vi "stations PING.vi"(5 "error in (no error)":errorcluster, 7 "Ping Timeout (ms)":i32=5000, 8 "IP Address":string) -> (0 "error out":errorcluster, 1 "Valid Test Station?":bool, 3 "PING Response":string)   [LabVIEW 2011]
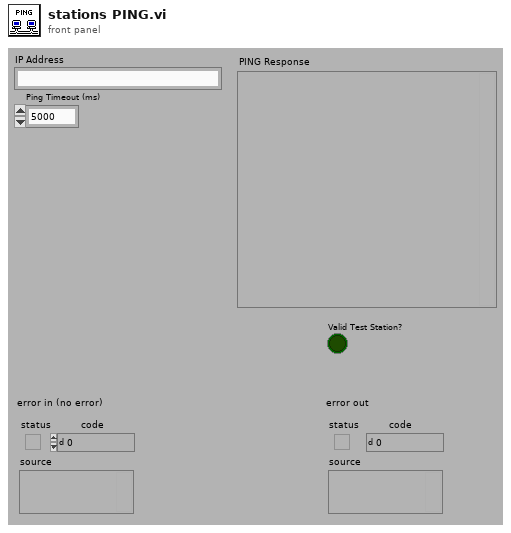
[diagram p1: front panel]
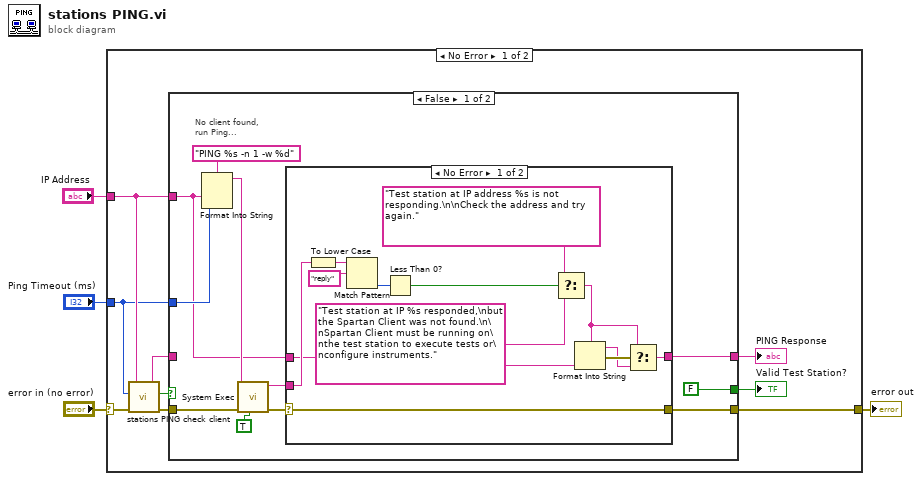
[diagram p0: block diagram]
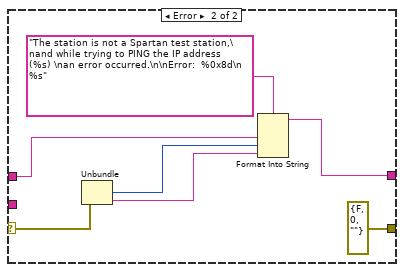
[diagram p2: hidden frame]
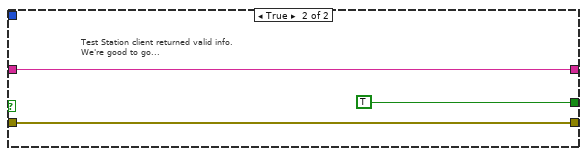
[diagram p3: hidden frame]
diagram:
  n1 = case shown="No Error" "error in (no error)" {
    selector: "error in (no error)" -> [w10 w48]
    tunnel: [w13 w48] -> w4
    tunnel: "Ping Timeout (ms)" -> [w6 _]
    tunnel: "IP Address" -> [w7 _]
    frame No Error {
      n2 = call "stations PING check client.vi"("error in (no error)"=w10, "Timeout, ms (10000)"=w6, "Client IP (\"\")"=w7) -> ("error out"=w5:errorcluster, "TestStation Client?"=w9:bool, "Response"=w8:string)  [unwired: 2 out]
      n3 = case shown="False" w9 {
        tunnel: [w19 w45] -> w13
        tunnel: [FALSE TRUE] -> w11
        tunnel: w7 -> [w16 _]
        tunnel: w8 -> [_ w47]
        tunnel: [w14 w47] -> w12
        tunnel: w6 -> [w17 _]
        tunnel: w5 -> [w15 w45]
        frame False {
          # "No client found,\nrun Ping..."
          n4 = Format Into String(format string="PING %s -n 1 -w %d" ("command line"), w16, w17) -> (resulting string=w22:string)  [unwired: 2 in, 1 out]
          n5 = call <vilib>:"System Exec.vi"("run minimized? (F)"=TRUE, "error in (no error)"=w15, "command line"=w22) -> ("error out"=w20:errorcluster, "standard output"=w18:string)  [unwired: 3 in, 4 out]
          n6 = case shown="No Error" w20 {
            selector: w20 -> [w29 w44]
            tunnel: [w29 errorcluster {"status"=FALSE, "code"=0, "source"=""} ("error IO")] -> w19
            tunnel: w18 -> [w37 _]
            tunnel: w16 -> [w33 w40]
            tunnel: [w30 w42] -> w14
            frame No Error {
              n7 = To Lower Case(string=w37) -> (all lower case string=w36:string)
              n8 = Match Pattern(string=w36, regular expression="reply") -> (offset past match=w34:i32)  [unwired: 4 out]
              n9 = Less Than 0?(x=w34) -> (x < 0?=w28:bool)
              n10 = Select(t="Test station at IP address %s is not responding.\n\nCheck the address and try again." ("source"), s=w28, f="Test station at IP %s responded,\nbut the Spartan Client was not found.\n\nSpartan Client must be running on\nthe test station to execute tests or\nconfigure instruments." ("source")) -> (s? t:f=w27:string)
              n11 = Format Into String(format string=w27, w33) -> (resulting string=w31:string, error out=w32:errorcluster)  [unwired: 2 in]
              n12 = Select(t=w27, s=w32, f=w31) -> (s? t:f=w30:string)
            }
            frame Error {
              n13 = Unbundle(w44) -> ("code"=w39:i32, "source"=w38:string)  [unwired: 1 out]
              n14 = Format Into String(format string="The station is not a Spartan test station,\nand while trying to PING the IP address (%s) \nan error occurred.\n\nError:  %0x8d\n %s" ("command line"), w40, w39, w38) -> (resulting string=w42:string)  [unwired: 2 in, 1 out]
            }
          }
        }
        frame True {
          # "Test Station client returned valid info.\nWe're good to go..."
        }
      }
      "PING Response" <- w12
      "Valid Test Station?" <- w11
    }
    frame Error {
    }
  }
  "error out" <- w4
